vi "water_subvi.vi"() -> (1 "Message":string, 2 "time":dbl, 3 "volume":dbl)   [LabVIEW 2019]
uses:
  <vilib>/Utility/file.llb/Read Delimited Spreadsheet (string).vi
panel:
  out "Recipe":string
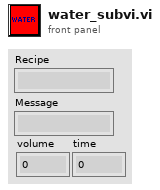
[diagram p1: front panel]
types:
  T1 = cluster{"Recipe":string, "Message":string, "volume":dbl, "time":dbl}
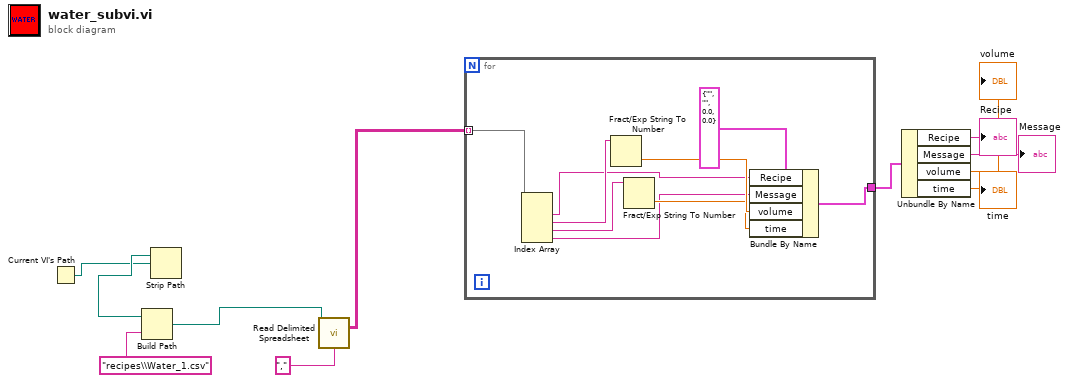
[diagram p0: block diagram]
diagram:
  n1 = Current VI's Path() -> (path=w2:path)
  n2 = Strip Path(path=w2) -> (stripped path=w4:path)  [unwired: 1 out]
  n3 = Build Path(base path=w4, name or relative path="recipes\\Water_1.csv") -> (appended path=w1:path)
  n4 = call-poly <vilib>:"Read Delimited Spreadsheet.vi"("file path (dialog if empty)"=w1, "delimiter (\\t)"="," ("delimiter (\\t)")) -> ("all rows"=w10:string[][])  [unwired: 8 in, 5 out]
  n5 = for {
    tunnel: w10 -> [w20] mode=indexing
    tunnel: [w12] -> w9
    n6 = Index Array(array=w20) -> (element #1=w13:string, element #2=w19:string, element #3=w16:string, element #4=w14:string)  [unwired: 4 in]
    n7 = Fract/Exp String To Number(string=w19) -> (number=w17:dbl)  [unwired: 3 in, 1 out]
    n8 = Fract/Exp String To Number(string=w16) -> (number=w15:dbl)  [unwired: 3 in, 1 out]
    n9 = Bundle By Name(cluster=T1 {"Recipe"="", "Message"="", "volume"=0.0, "time"=0.0} ("Receipes"), "Recipe"=w13, "Message"=w14, "volume"=w17, "time"=w15) -> (w12:T1)
  }
  n10 = Unbundle By Name(w9) -> ("Recipe"=→"Recipe":string, "Message"=→"Message":string, "volume"=→"volume":dbl, "time"=→"time":dbl)
